vi "Choreo_Util_AllianceFlipHeading.vi"(11 "heading":dbl) -> (3 "FlippedHeading":dbl)   [LabVIEW 2019, in "ChoreoLib.lvlib"]
doc: "trajectory, mirrored across the field midline.\n\nInputs: \n - ChoreoTrajectory - cluster - Input trajectory\n\nOutputs:\n - Flipped Trajectory - cluster - trajectory, mirrored across the field midline."
uses:
  ChoreoLib.lvlib
  Choreo_Choreo_Globals.vi
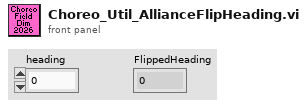
[diagram p1: front panel]
types:
  T1 = typedef "ChoreoLib.lvlib/Choreo_Util_AllianceFlipType.ctl" = enum16{"MIRRORED", "ROTATE_AROUND"}
  T2 = cluster{"Year":i32, "AllianceFlipType":T1, "FieldLength":dbl, "FieldWidth":dbl}
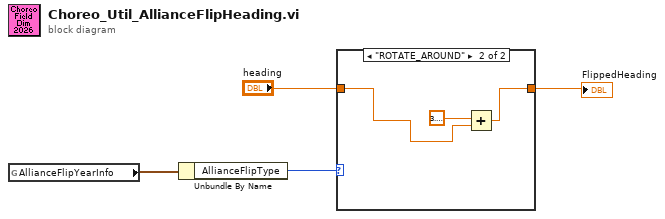
[diagram p0: block diagram]
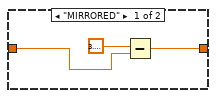
[diagram p2: hidden frame]
diagram:
  n1 = global read "Choreo_Choreo_Globals.vi" "AllianceFlipYearInfo"() -> (w4:T2)
  n2 = Unbundle By Name(w4) -> ("AllianceFlipType"=w3:T1)
  n3 = case shown="\"ROTATE_AROUND\"" w3 {
    tunnel: "heading" -> [w6 w9]
    tunnel: [w5 w8] -> w1
    frame "MIRRORED" {
      n4 = Subtract(x=3.141592653589793, y=w6) -> (x-y=w5:dbl)
    }
    frame "ROTATE_AROUND" {
      n5 = Add(x=3.141592653589793, y=w9) -> (x+y=w8:dbl)
    }
  }
  "FlippedHeading" <- w1
